vi "AES Calculate Replay Address.vi"(7 "AngleToAddress":fxp<+,18,7> format="%.14g", 8 "Offset (0)":fxp<+/-,61,10>, 9 "Crank Angle":fxp<+,60,9> format="%.54g", 10 "CycleAngle?":bool, 11 "Cycle Angle":fxp<+,61,10>) -> (3 "memory address":u32)   [LabVIEW 2010, in "AES.lvlib" / "AES FPGA.lvlib"]
doc: "This IP applies an adjustable offset to the crank or cycle angle to provide VVT functionality for data replay. It then multiplies the engine angle by the angle to address scalar to determine what memory address to look up for data replay."
uses:
  AES FPGA.lvlib
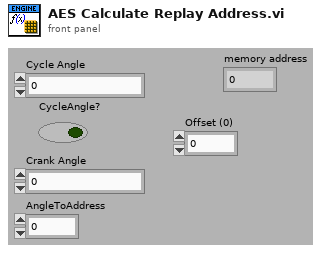
[diagram p1: front panel]
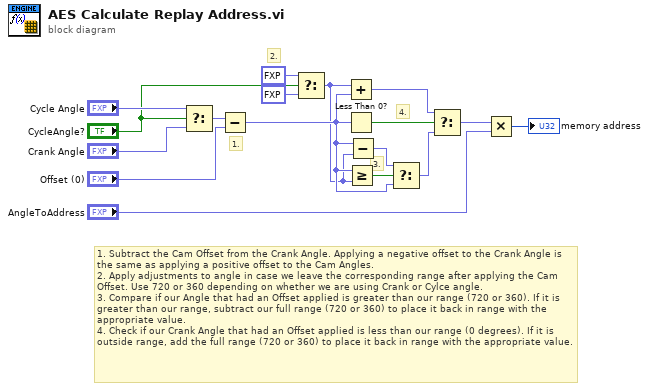
[diagram p0: block diagram]
diagram:
  # "1. Subtract the Cam Offset from the Crank Angle. Applying a negative offset to the Crank Angle is the same as applying a positive offset to the Cam Angles.\n2. Apply adjustments to angle in case we leave the corresponding range after applying the Cam Offset. Use 720 or 360 depending on whether we are using Crank or Cylce angle.\n3. Compare if our Angle that had an Offset applied is greater than our range (720 or 360). If it is greater than our range, subtract our full range (720 or 360) to place it back in range with the appropriate value.\n4. Check if our Crank Angle that had an Offset applied is less than our range (0 degrees). If it is outside range, add the full range (720 or 360) to place it back in range with the appropriate value."
  # "4."
  # "3."
  # "2."
  # "1."
  n1 = Select(t="Cycle Angle", s="CycleAngle?", f="Crank Angle") -> (s? t:f=w5:fxp<+,61,10>)
  n2 = Subtract(x=w5, y="Offset (0)") -> (x-y=w12:fxp<+/-,63,12>)
  n3 = Select(t=fxp<+,7,10> 720.0 ("x"), s="CycleAngle?", f=fxp<+,6,9> 360.0 ("x")) -> (s? t:f=w8:fxp<+,7,10>)
  n4 = Add(x=w8, y=w12) -> (x+y=w15:fxp<+/-,64,13>)
  n5 = Less Than 0?(x=w12) -> (x < 0?=w16:bool)
  n6 = Greater Or Equal?(x=w12, y=w8) -> (x >= y?=w14:bool)
  n7 = Subtract(x=w12, y=w8) -> (x-y=w13:fxp<+/-,63,12>)
  n8 = Select(t=w13, s=w14, f=w12) -> (s? t:f=w11:fxp<+/-,63,12>)
  n9 = Select(t=w15, s=w16, f=w11) -> (s? t:f=w3:fxp<+/-,64,13>)
  n10 = Multiply(x=w3, y="AngleToAddress") -> (x*y=→"memory address":u32)
